vi "CAN Message Recieve Rate.vi"() -> ()   [LabVIEW 2014]
panel:
  out "Elapsed Time":dbl
  out "Messages/second":dbl
  in  "x":bool
  out "error out":errorcluster
  out "index":i32
  in  "baud rate (125000 bps)":u32=1000000
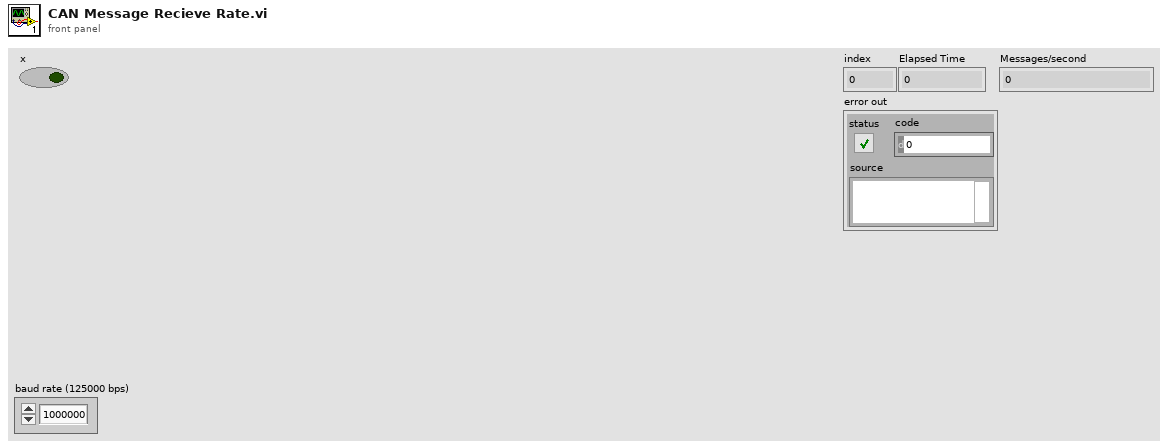
[diagram p1: front panel]
types:
  T1 = typedef "CANFrameControl.ctl" = cluster{"identifier":u32, "extended?":bool, "type":u8, "payload":u8[]}
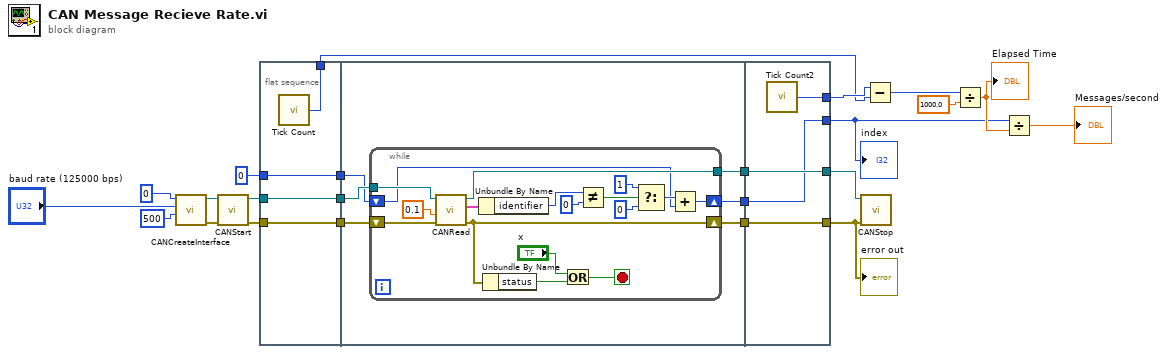
[diagram p0: block diagram]
diagram:
  n1 = call <vilib>:"CANCreateInterface.vi"("receive queue size (5)"=u32 500, "baud rate (125000 bps)"="baud rate (125000 bps)", "interface index"=u32 0) -> ("error out"=w23:errorcluster, "interface object out"=w22:refnum<k20>)  [unwired: 7 in]
  n2 = call <vilib>:"CANStart.vi"("error in (no error)"=w23, "interface object in"=w22) -> ("error out"=w15:errorcluster, "interface object out"=w21:refnum<k20>)  [unwired: 8 in]
  n3 = flat-sequence {
    tunnel: w15 -> [w25]
    tunnel: 0 ("index") -> [w26]
    tunnel: w21 -> [w27]
    tunnel: [w27] -> w8
    tunnel: [w26] -> w7
    tunnel: [w25] -> w6
    tunnel: [w24] -> w1
    tunnel: w8 -> [w33]
    tunnel: w7 -> [w30]
    tunnel: w6 -> [w29]
    tunnel: [w32] -> w5
    tunnel: [w31] -> w4
    tunnel: [w28] -> w3
    tunnel: [w52] -> w10
    tunnel: [w53] -> w19
    tunnel: [w54] -> w20
    tunnel: w5 -> [w54]
    tunnel: w4 -> [w53]
    tunnel: w3 -> [w52]
    tunnel: [w51] -> w2
    frame #0 {
      n4 = call "Tick Count"() -> ("Tick Count(mSec)"=w24:u32)
    }
    frame #1 {
      n5 = while {
        tunnel: w33 -> [w50]
        tunnel: [w49] -> w32
        shift-right: [w38] -> w28
        shift-left: w30 -> [w36]
        shift-right: [w45] -> w31
        shift-left: w29 -> [w46]
        stop <- w44 stop-if-true
        n6 = call <vilib>:"CANRead.vi"("error in (no error)"=w46, "timeout (0 s)"=0.1, "interface object in"=w50) -> ("error out"=w45:errorcluster, "CAN frame"=w48:T1, "interface object out"=w49:refnum<k20>)  [unwired: 5 in, 1 out]
        n7 = Unbundle By Name(w48) -> ("identifier"=w41:u32)
        n8 = Unbundle By Name(w45) -> ("status"=w43:bool)
        n9 = Or(x="x", y=w43) -> (x .or. y?=w44:bool)
        n10 = Not Equal?(x=w41, y=u32 0) -> (x != y?=w39:bool)
        n11 = Select(t=1, s=w39, f=0 ("index")) -> (s? t:f=w37:i32)
        n12 = Add(x=w37, y=w36) -> (x+y=w38:i32)
      }
    }
    frame #2 {
      n13 = call "Tick Count2"() -> ("Tick Count(mSec)"=w51:u32)
    }
  }
  n14 = call <vilib>:"CANStop.vi"("error in (no error)"=w19, "interface object in"=w20) -> ()  [unwired: 8 in, 2 out]
  n15 = Subtract(x=w2, y=w1) -> (x-y=w13:u32)
  n16 = Divide(x=w13, y=1000.0) -> (x/y=w11:dbl)
  "Elapsed Time" <- w11
  n17 = Divide(x=w10, y=w11) -> (x/y=→"Messages/second":dbl)
  "index" <- w10
  "error out" <- w19
